vi "Insert Child Attributes.vi"(7 "Actor in":refnum<class "Actor.lvclass">, 10 "Child Attributes":refnum<class "Attributes.lvclass">) -> (5 "Actor out":refnum<class "Actor.lvclass">)   [LabVIEW 2025, in "jettl.lvlib"]
uses:
  jettl.lvlib
  Attributes/Attributes.lvclass
  Actor/Actor.lvclass
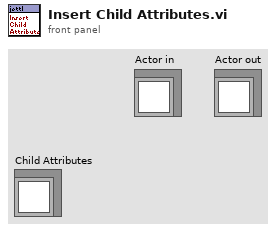
[diagram p1: front panel]
types:
  T1 = typedef "jettl.lvlib/All Child Attributes.ctl" = map{string, refnum<class "Attributes.lvclass">}
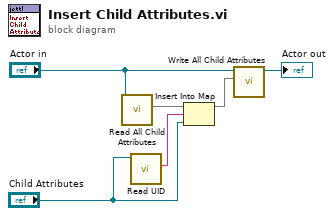
[diagram p0: block diagram]
diagram:
  n1 = call-dynamic "Read All Child Attributes.vi"("Actor in"="Actor in") -> ("All Child Attributes"=w1:T1)  [unwired: 10 in]
  n2 = call-dynamic "Read UID.vi"("Attributes in"="Child Attributes") -> ("UID"=w5:string)  [unwired: 10 in]
  n3 = Insert Into Map(map in=w1, key=w5, value="Child Attributes") -> (map out=w2:T1)  [unwired: 2 out]
  n4 = call-dynamic "Write All Child Attributes.vi"("All Child Attributes"=w2, "Actor in"="Actor in") -> ("Actor out"=→"Actor out":refnum<class "Actor.lvclass">)  [unwired: 9 in]
